vi "lvssh2_abstract_init.vi"(8 "error in (no error)":errorcluster, 10 "lvssh2_session_callback_receive":refnum<vi>, 11 "lvssh2_session_callback_send":refnum<vi>) -> (0 "error out":errorcluster, 2 "event callback refnum":refnum<k27>, 3 "abstract":T1)   [LabVIEW 2013, in "libssh2.lvlib"]
doc: "Initialize abstract for lvssh2."
uses:
  libssh2.lvlib
  lvssh2_abstract.ctl
  lvssh2_session_callback_send_function_input_args_32.ctl
  lvssh2_session_callback_receive_function_input_args_32.ctl
  lvssh2_session_callback_receive_handler_32.vi
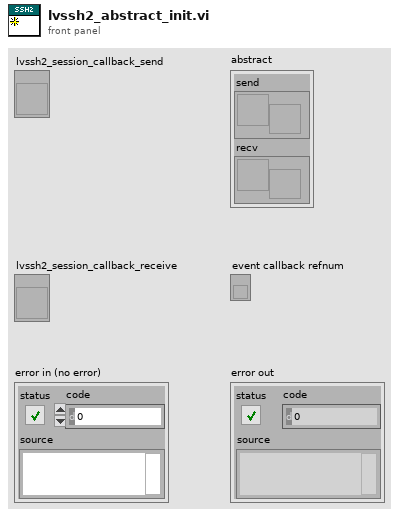
[diagram p1: front panel]
types:
  T1 = typedef "libssh2.lvlib/lvssh2_abstract.ctl" = cluster{"send":refnum<user-event>, "recv":refnum<user-event>}
  T2 = typedef "libssh2.lvlib/lvssh2_session_callback_receive_function_input_args_32.ctl" = cluster{"socket":u32, "buffer":u32, "length":u32, "flags":i32}
  T3 = typedef "libssh2.lvlib/lvssh2_session_callback_send_function_input_args_32.ctl" = cluster{"socket":u32, "buffer":u32, "length":u32, "flags":i32}
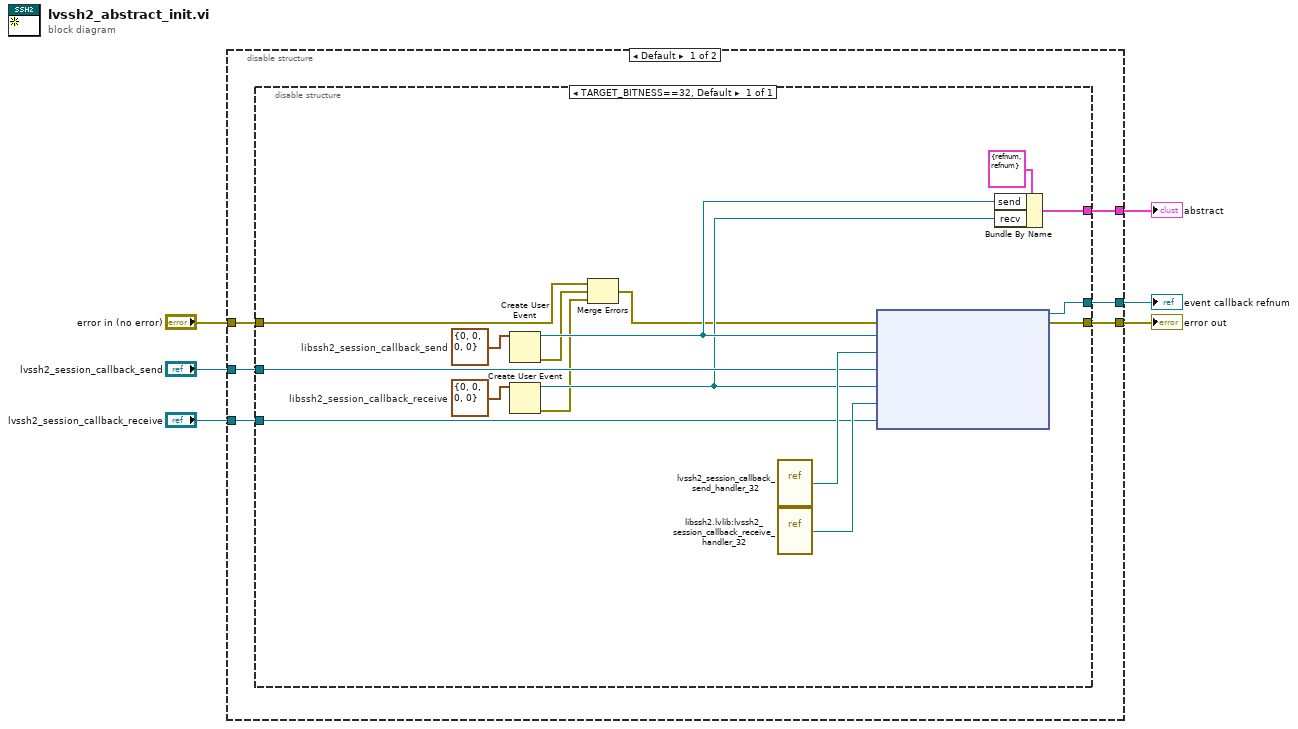
[diagram p0: block diagram]
diagram:
  n1 = disable-structure shown="Default" {
    disable-tunnel: [w12 w29] -> w6
    disable-tunnel: "error in (no error)" -> [w11 w29]
    disable-tunnel: [w10 _] -> w4
    disable-tunnel: [w9 _] -> w3
    disable-tunnel: "lvssh2_session_callback_send" -> [w8 _]
    disable-tunnel: "lvssh2_session_callback_receive" -> [w7 _]
    frame condition #0 (active) {
      n2 = disable-structure shown="TARGET_BITNESS==32, Default" {
        disable-tunnel: [w22] -> w12
        disable-tunnel: w11 -> [w16]
        disable-tunnel: [w28] -> w10
        disable-tunnel: [w21] -> w9
        disable-tunnel: w8 -> [w23]
        disable-tunnel: w7 -> [w18]
        frame condition #0 (active) {
          w20 = T2 {"socket"=0, "buffer"=0, "length"=0, "flags"=0}  # libssh2_session_callback_receive
          w25 = T3 {"socket"=0, "buffer"=0, "length"=0, "flags"=0}  # libssh2_session_callback_send
          n3 = Create User Event(user event datatype=w25) -> (user event=w24:refnum<user-event>, error out=w15:errorcluster)  [unwired: 1 in]
          n4 = Create User Event(user event datatype=w20) -> (user event=w17:refnum<user-event>, error out=w14:errorcluster)  [unwired: 1 in]
          n5 = Merge Errors(w16, w15, w14) -> (w13:errorcluster)
          n6 = vi-ref "lvssh2_session_callback_send_handler_32.vi"() -> ("vi reference"=w26:refnum<vi>)
          n7 = vi-ref "libssh2.lvlib:lvssh2_session_callback_receive_handler_32.vi"() -> ("vi reference"=w19:refnum<vi>)
          n8 = node(w13, w24, w26, w23, w17, w19, w18) -> (w21:refnum<k27>, w22:errorcluster)  [unwired: 1 in]
          n9 = Bundle By Name(cluster=T1 {"send"=refnum, "recv"=refnum} ("abstract"), "send"=w24, "recv"=w17) -> (w28:T1)
        }
      }
    }
    frame condition #1 {
    }
  }
  "error out" <- w6
  "abstract" <- w4
  "event callback refnum" <- w3
